vi "Replace Debug Log History Method.vi"(8 "error in (no error)":errorcluster, 11 "CSM-Helper in":refnum<class "CSM-Helper.lvclass">) -> (0 "error out":errorcluster, 3 "CSM-Helper out":refnum<class "CSM-Helper.lvclass">)   [LabVIEW 2017, in "CSM-Helper.lvclass"]
uses:
  CSM-Helper.lvclass
  CSM-Helper.lvclass/CSM-Helper.ctl
  Properties/Read Parse State Queue Ref.vi
  Utility/_Support/SubVI.llb/csmHelper-SubVI.lvlib
  Utility/_Support/Terminals.llb/csmHelper-Terminals.lvlib
  _Shared/CSM Shared.lvlib
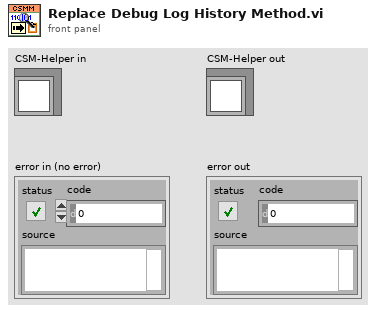
[diagram p1: front panel]
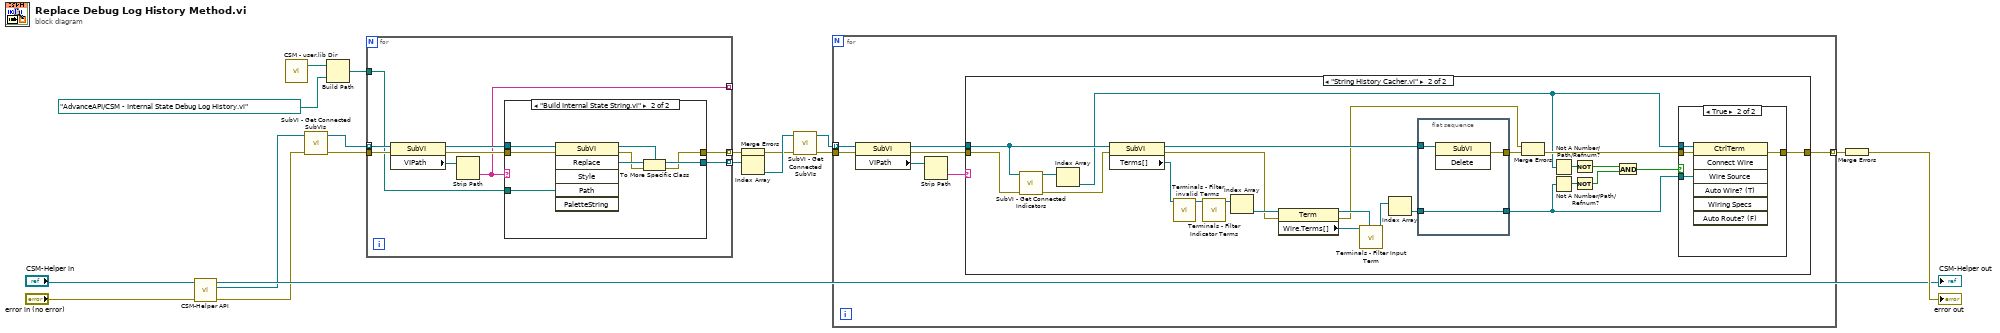
[diagram p0: block diagram]
diagram:
  n1 = call-poly "CSM-Helper API.vi"("error in (no error)"="error in (no error)", "CSM-Helper in"="CSM-Helper in") -> ("error out"=w3:errorcluster, "Parse State Queue"=w4:refnum<vi>, "CSM-Helper out"=→"CSM-Helper out":refnum<class "CSM-Helper.lvclass">)  [unwired: 7 in]
  n2 = call "CSM - user.lib Dir.vi"() -> ("csm_user.lib_dir"=w8:path)  [unwired: 2 in, 1 out]
  n3 = call "SubVI - Get Connected SubVIs.vi"("error in (no error)"=w3, "SubVI in"=w4) -> ("error out"=w7:errorcluster, "Array"=w6:refnum<vi>[])  [unwired: 8 in]
  n4 = Build Path(base path=w8, name or relative path=path "AdvanceAPI/CSM - Internal State Debug Log History.vi") -> (appended path=w10:path)
  n5 = for {
    tunnel: w6 -> [w27] mode=indexing
    tunnel: [w22] -> _ mode=indexing
    tunnel: w7 -> [w24]
    tunnel: w10 -> [w21]
    tunnel: [w20] -> w11 mode=indexing
    tunnel: [w19] -> w12 mode=indexing
    n6 = property class="SubVI"(reference=w27, error in=w24) -> (reference out=w25:refnum<vi>, error out=w23:errorcluster, "VIPath"=w26:path)
    n7 = Strip Path(path=w26) -> (name=w22:string)  [unwired: 1 out]
    n8 = case shown="\"Build Internal State String.vi\"" w22 {
      tunnel: w25 -> [_ w36]
      tunnel: w23 -> [w28 w35]
      tunnel: w21 -> [_ w34]
      tunnel: [w28 w29] -> w20
      tunnel: [_ w32] -> w19
      frame "False", Default {
      }
      frame "Build Internal State String.vi" {
        n9 = invoke class="SubVI" method="Replace"(reference=w36, error in=w35, "Path"=w34) -> (reference out=w33:refnum<vi>, error out=w30:errorcluster, "Replace"=w31:refnum<vi>)  [unwired: 3 in, 3 out]
        n10 = To More Specific Class(target class=w33, reference=w31, error in=w30) -> (specific class reference=w32:refnum<vi>, error out=w29:errorcluster)
      }
    }
  }
  n11 = Merge Errors(w11) -> (w15:errorcluster)
  n12 = Index Array(array=w12) -> (element=w18:refnum<vi>)  [unwired: 1 in]
  n13 = call "SubVI - Get Connected SubVIs.vi"("error in (no error)"=w15, "SubVI in"=w18) -> ("error out"=w16:errorcluster, "Array"=w17:refnum<vi>[])  [unwired: 8 in]
  n14 = for {
    tunnel: w17 -> [w43] mode=indexing
    tunnel: w16 -> [w40]
    tunnel: [w37] -> w13 mode=indexing
    n15 = property class="SubVI"(reference=w43, error in=w40) -> (reference out=w41:refnum<vi>, error out=w39:errorcluster, "VIPath"=w42:path)
    n16 = Strip Path(path=w42) -> (name=w38:string)  [unwired: 1 out]
    n17 = case shown="\"String History Cacher.vi\"" w38 {
      tunnel: w41 -> [_ w65]
      tunnel: w39 -> [w44 w69]
      tunnel: [w44 w66] -> w37
      frame "False", Default {
      }
      frame "String History Cacher.vi" {
        n18 = call "SubVI - Get Connected Indicators.vi"("error in (no error)"=w69, "SubVI in"=w65) -> ("error out"=w59:errorcluster, "Array 2"=w68:refnum<vi>[])  [unwired: 8 in]
        n19 = Index Array(array=w68) -> (element=w51:refnum<vi>)  [unwired: 1 in]
        n20 = property class="SubVI"(reference=w65, error in=w59) -> (reference out=w64:refnum<vi>, error out=w54:errorcluster, "Terms[]"=w62:refnum<vi>[])
        n21 = call "Terminals - Filter invalid Terms.vi"("Terms[]"=w62) -> ("Terms[] out"=w61:refnum<vi>[])  [unwired: 10 in]
        n22 = call "Terminals - Filter Indicator Terms.vi"("Terms[]"=w61) -> ("Terms[] out"=w63:refnum<vi>[])  [unwired: 10 in]
        n23 = Index Array(array=w63) -> (element=w60:refnum<vi>)  [unwired: 1 in]
        n24 = property class="Term"(reference=w60, error in=w54) -> (reference out=w57:refnum<vi>, error out=w52:errorcluster, "Wire.Terms[]"=w58:refnum<vi>[])
        n25 = call "Terminals - Filter Input Term.vi"("InnerTerminal in"=w57, "Wire.Terms[] in"=w58) -> ("Wire.Terms[] out"=w55:refnum<vi>[])  [unwired: 9 in]
        n26 = Index Array(array=w55) -> (element=w56:refnum<vi>)  [unwired: 1 in]
        n27 = flat-sequence {
          tunnel: [w77] -> w67
          tunnel: w64 -> [w76]
          tunnel: [w75] -> w50
          tunnel: w56 -> [w75]
          frame #0 {
            n28 = invoke class="SubVI" method="Delete"(reference=w76) -> (error out=w77:errorcluster)  [unwired: 2 in, 2 out]
          }
        }
        n29 = Merge Errors(w52, w67) -> (w53:errorcluster)
        n30 = Not A Number/Path/Refnum?(number/path/refnum=w51) -> (NaN/Path/Refnum?=w49:bool)
        n31 = Not A Number/Path/Refnum?(number/path/refnum=w50) -> (NaN/Path/Refnum?=w48:bool)
        n32 = Not(x=w49) -> (.not. x?=w46:bool)
        n33 = Not(x=w48) -> (.not. x?=w47:bool)
        n34 = And(x=w46, y=w47) -> (x .and. y?=w45:bool)
        n35 = case shown="True" w45 {
          tunnel: [w70 w74] -> w66
          tunnel: w53 -> [w70 w73]
          tunnel: w51 -> [_ w72]
          tunnel: w50 -> [_ w71]
          frame False {
          }
          frame True {
            n36 = invoke class="CtrlTerm" method="Connect Wire"(reference=w72, error in=w73, "Wire Source"=w71) -> (error out=w74:errorcluster)  [unwired: 4 in, 6 out]
          }
        }
      }
    }
  }
  n37 = Merge Errors(w13) -> (→"error out":errorcluster)
